vi "Delta robot inverse kinematic.vi"(4 "re":dbl=224.0 format="%#_13g", 5 "rf":dbl=144.0 format="%#_13g", 6 "e":dbl=39.092 format="%#_13g", 7 "f":dbl=63.127 format="%#_13g", 8 "z0":dbl format="%#_13g", 9 "y0":dbl format="%#_13g", 10 "x0":dbl format="%#_13g") -> (0 "thetaZ":dbl, 1 "thetaY":dbl, 2 "thetaX":dbl, 3 "non-existing point":bool)   [LabVIEW 2019]
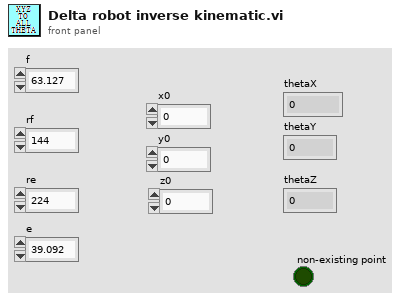
[diagram p1: front panel]
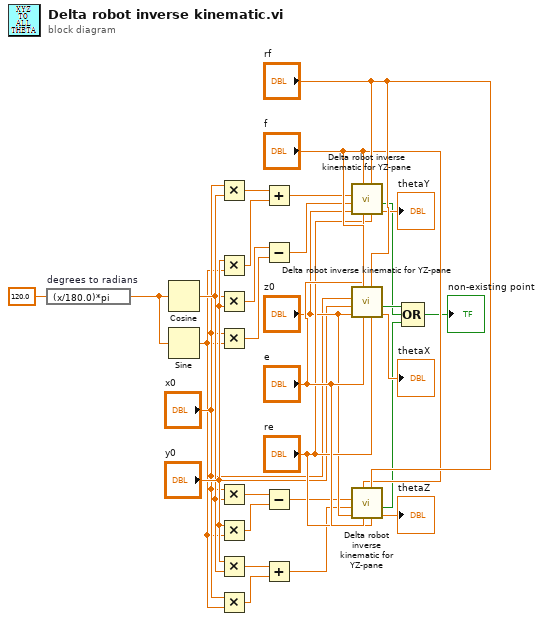
[diagram p0: block diagram]
diagram:
  n1 = expression code="(x/180.0)*pi" "degrees to radians"(120.0) -> (w16:dbl)
  n2 = Cosine(x=w16) -> (cos(x)=w4:dbl)
  n3 = Sine(x=w16) -> (sin(x)=w2:dbl)
  n4 = Multiply(x="x0", y=w4) -> (x*y=w17:dbl)
  n5 = Multiply(x="y0", y=w2) -> (x*y=w15:dbl)
  n6 = Multiply(x=w4, y="y0") -> (x*y=w13:dbl)
  n7 = Multiply(x="x0", y=w2) -> (x*y=w12:dbl)
  n8 = Multiply(x="x0", y=w4) -> (x*y=w9:dbl)
  n9 = Multiply(x="y0", y=w2) -> (x*y=w10:dbl)
  n10 = Multiply(x="y0", y=w4) -> (x*y=w7:dbl)
  n11 = Multiply(x="x0", y=w2) -> (x*y=w8:dbl)
  n12 = Add(x=w17, y=w15) -> (x+y=w14:dbl)
  n13 = Subtract(x=w13, y=w12) -> (x-y=w11:dbl)
  n14 = Subtract(x=w9, y=w10) -> (x-y=w6:dbl)
  n15 = Add(x=w7, y=w8) -> (x+y=w1:dbl)
  n16 = call "Delta robot inverse kinematic for YZ-pane.vi"("re"="re", "rf"="rf", "e"="e", "f"="f", "z0"="z0", "y0"=w11, "x0"=w14) -> ("theta"=→"thetaY":dbl, "non-existing point"=w20:bool)  [unwired: 3 in]
  n17 = call "Delta robot inverse kinematic for YZ-pane.vi"("re"="re", "rf"="rf", "e"="e", "f"="f", "z0"="z0", "y0"="y0", "x0"="x0") -> ("theta"=→"thetaX":dbl, "non-existing point"=w21:bool)  [unwired: 3 in]
  n18 = call "Delta robot inverse kinematic for YZ-pane.vi"("re"="re", "rf"="rf", "e"="e", "f"="f", "z0"="z0", "y0"=w1, "x0"=w6) -> ("theta"=→"thetaZ":dbl, "non-existing point"=w19:bool)  [unwired: 3 in]
  n19 = Compound Arithmetic op=OR(w21, w20, w19) -> (→"non-existing point":bool)
